vi "main(Manual_Voltage_Log_Analysis).vi"() -> ()   [LabVIEW 2015]
uses:
  <vilib>/Analysis/baseanly.llb/Mean (DBL).vi
  <vilib>/Analysis/NI_AALBase.lvlib
panel:
  in  "file path (use dialog)":path
  out "파일 이름":string[](array[string])
  out "Battery":u32[][](array[numeric])
  out "Avg":dbl[][](array[numeric])
  in  "Number of Sample for avg.":i32
  in  "Number of Data Down-Sampling":i32
  in  "File Path":path
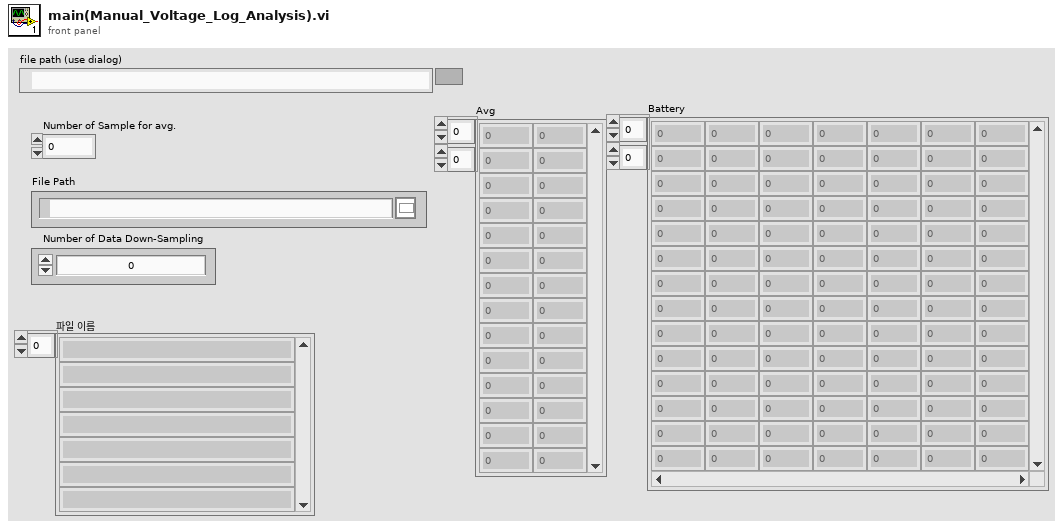
[diagram p1: front panel]
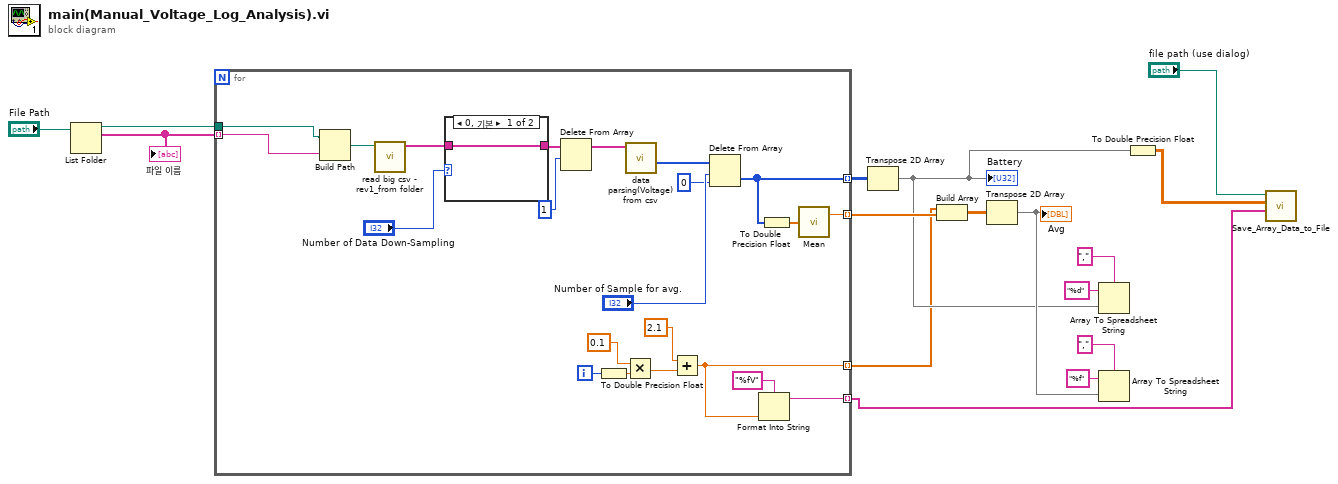
[diagram p0: block diagram]
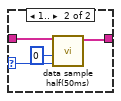
[diagram p2: hidden frame]
diagram:
  n1 = List Folder(path="File Path") -> (path out=w16:path, filenames=w14:string[])  [unwired: 3 in, 2 out]
  "파일 이름" <- w14
  n2 = for {
    tunnel: w16 -> [w29]
    tunnel: w14 -> [w28] mode=indexing
    tunnel: [w27] -> w13 mode=indexing
    tunnel: [w25] -> w8 mode=indexing
    tunnel: [w18] -> w2 mode=indexing
    tunnel: [w17] -> w1 mode=indexing
    i -> [w24]
    n3 = Build Path(base path=w29, name or relative path=w28) -> (appended path=w38:path)
    n4 = call "read big csv - rev1_from folder.vi"("파일 경로(대화 상자 사용)"=w38) -> ("배열"=w37:string[])  [unwired: 10 in]
    n5 = case shown="0, 기본" "Number of Data Down-Sampling" {
      selector: "Number of Data Down-Sampling" -> [_ w42]
      tunnel: w37 -> [w39 w43]
      tunnel: [w39 w41] -> w35
      frame 0, Default {
      }
      frame 1.. {
        n6 = call "data sample half(50ms).vi"("Number of Remove data"=w42, "Offset"=0, "Array"=w43) -> ("Array out"=w41:string[])  [unwired: 8 in]
      }
    }
    n7 = Delete From Array(array=w35, length=1 ("길이")) -> (array with subset deleted=w33:string[])  [unwired: 1 in, 1 out]
    n8 = To Double Precision Float(number=w24) -> (double precision float=w22:dbl)
    n9 = Multiply(x=0.1, y=w22) -> (x*y=w21:dbl)
    n10 = call "data parsing(Voltage) from csv.vi"("배열"=w33) -> ("Battery"=w32:u32[])  [unwired: 7 in, 3 out]
    n11 = Add(x=2.1, y=w21) -> (x+y=w18:dbl)
    n12 = Delete From Array(array=w32, length="Number of Sample for avg.", index=0 ("인덱스")) -> (deleted portion=w27:u32[])  [unwired: 1 out]
    n13 = Format Into String(format string="%fV" ("포맷 문자열"), w18) -> (resulting string=w17:string)  [unwired: 2 in, 1 out]
    n14 = To Double Precision Float(number=w27) -> (double precision float=w26:dbl[])
    n15 = call-poly <vilib>:"Mean.vi"("X"=w26) -> ("mean"=w25:dbl)  [unwired: 1 out]
  }
  n16 = Transpose 2D Array(2D array=w13) -> (transposed array=w4:u32[][])
  "Battery" <- w4
  n17 = Build Array(w2, w8) -> (w7:dbl[][])
  n18 = Transpose 2D Array(2D array=w7) -> (transposed array=w6:dbl[][])
  "Avg" <- w6
  n19 = Array To Spreadsheet String(delimiter (Tab)="," ("구분 문자(탭)"), array=w4, 3:"%d" ("포맷 문자열")) -> ()  [unwired: 1 out]
  n20 = Array To Spreadsheet String(delimiter (Tab)="," ("구분 문자(탭)"), array=w6, 3:"%f" ("포맷 문자열")) -> ()  [unwired: 1 out]
  n21 = To Double Precision Float(number=w4) -> (double precision float=w3:dbl[][])
  n22 = call "Save_Array_Data_to_File.vi"("Header Array"=w1, "Array"=w3, "file path (use dialog)"="file path (use dialog)") -> ()  [unwired: 8 in, 1 out]
